vi "Data to String.vi"(7 "Precision (2)":i16=2, 10 "Data":dbl) -> (2 "String Data":string)   [LabVIEW 2013]
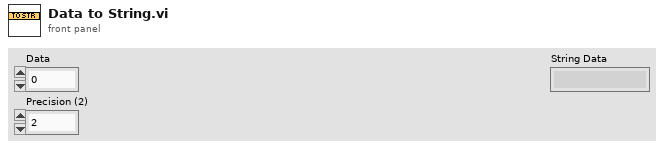
[diagram p1: front panel]
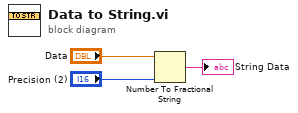
[diagram p0: block diagram]
diagram:
  n1 = Number To Fractional String(number="Data", precision (6)="Precision (2)") -> (F-format string=→"String Data":string)  [unwired: 2 in]
